vi "S2C_ExeScriptIndex.vi"(7 "Index":i32, 8 "Error In":errorcluster, 11 "IncRow?":bool) -> (0 "Error Out":errorcluster, 3 "TopCell Out":T1)   [LabVIEW 2015]
doc: "Determines the top row to display for auto-scrolling, and checks for the presents of a breakpoint."
uses:
  <vilib>/Utility/miscctls.llb/LVRowAndColumnUnsignedTypeDef.ctl
  Globals/S2C_Globals.vi
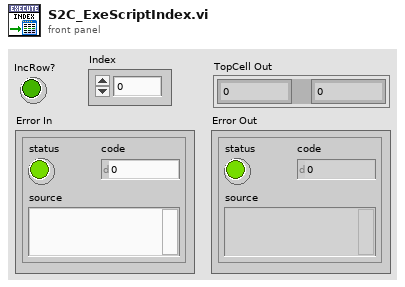
[diagram p1: front panel]
types:
  T1 = typedef "LVRowAndColumnUnsignedTypeDef.ctl" = cluster{"Row":u32, "Column":u32}
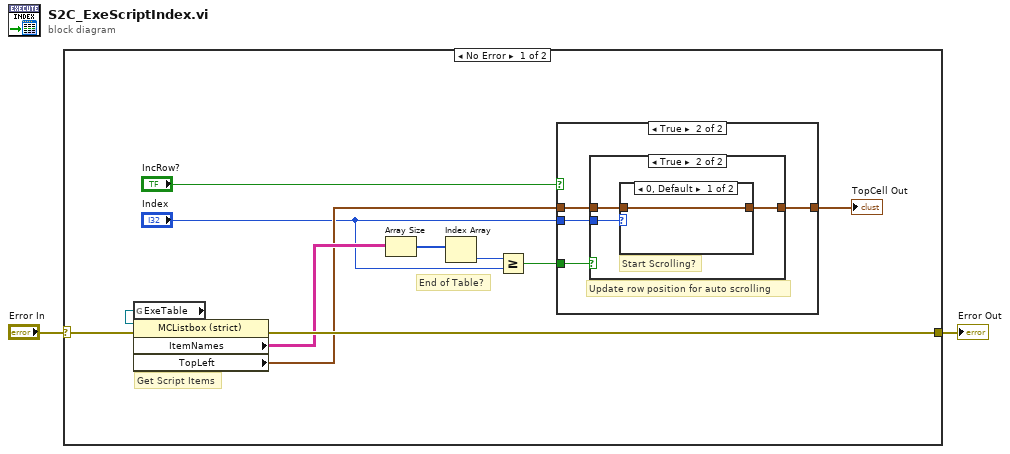
[diagram p0: block diagram]
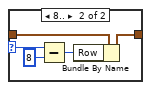
[diagram p4: hidden frame]
diagram:
  n1 = case shown="No Error" "Error In" {
    selector: "Error In" -> [w13 w29]
    tunnel: [w12 w29] -> w1
    frame No Error {
      # "Get Script Items"
      # "End of Table?"
      n2 = global read "S2C_Globals.vi" "ExeTable"() -> (w7:refnum<vi>)
      n3 = property class="MCListbox (strict)"(reference=w7, error in=w13) -> (error out=w12:errorcluster, "ItemNames"=w6:string[][], "TopLeft"=w5:T1)  [unwired: 1 out]
      n4 = Array Size(array=w6) -> (size(s)=w10:i32[])
      n5 = Index Array(array=w10) -> (element=w11:i32)  [unwired: 1 in]
      n6 = Greater Or Equal?(x=w11, y="Index") -> (x >= y?=w9:bool)
      n7 = case shown="True" "IncRow?" {
        tunnel: w9 -> [_ w18]
        tunnel: [w14 w17] -> w8
        tunnel: w5 -> [w14 w16]
        tunnel: "Index" -> [_ w15]
        frame False {
          # "Don't increment Row"
        }
        frame True {
          # "Update row position for auto scrolling"
          n8 = case shown="True" w18 {
            tunnel: w16 -> [w19 w22]
            tunnel: [w19 w21] -> w17
            tunnel: w15 -> [_ w20]
            frame False {
            }
            frame True {
              # "Start Scrolling?"
              n9 = case shown="0, Default" w20 {
                selector: w20 -> [_ w26]
                tunnel: w22 -> [w23 w28]
                tunnel: [w23 w27] -> w21
                frame 0, Default {
                }
                frame 8.. {
                  n10 = Subtract(x=w26, y=8) -> (x-y=w25:i32)
                  n11 = Bundle By Name(cluster=w28, "Row"=w25) -> (w27:T1)
                }
              }
            }
          }
        }
      }
      "TopCell Out" <- w8
    }
    frame Error {
    }
  }
  "Error Out" <- w1
